vi "Set Phase Ref.vi"(0 "VISA Resource Name":refnum<visa-resource-name>, 11 "error in (no error)":errorcluster {"code" format="%.0x"}) -> (4 "VISA Resource Name Out":refnum<visa-resource-name>, 15 "error out":errorcluster {"code" format="%.0x"})   [LabVIEW 2012, in "Agilent ESG Series.lvlib"]
doc: "This VI is sets the current output phase as zero reference.\nPhase adjustments are then set as relative to this zero reference."
uses:
  <instrlib>/Agilent ESG Series/Agilent ESG Series.lvlib
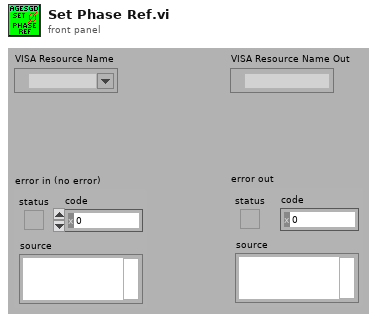
[diagram p1: front panel]
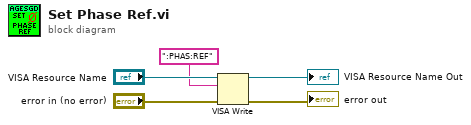
[diagram p0: block diagram]
diagram:
  n1 = VISA Write(VISA resource name="VISA Resource Name", write buffer=":PHAS:REF", error in (no error)="error in (no error)") -> (VISA resource name out=→"VISA Resource Name Out":refnum<visa-resource-name>, error out=→"error out":errorcluster)  [unwired: 1 out]
